vi "WinCI Run Provider.vi"(8 "error in (no error)":errorcluster) -> (0 "error out":errorcluster)   [LabVIEW 2017, in "NI_SCC_WinCI.lvlib"]
uses:
  <vilib>/SourceControl/Providers/WinCI/NI_SCC_WinCI.lvlib
  <vilib>/SourceControl/support/SCCSup Message Strings GLBL.vi
panel:
  out "result":i32
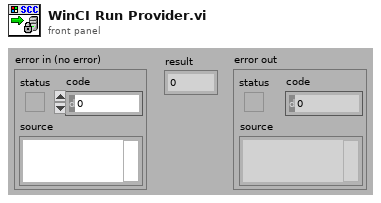
[diagram p1: front panel]
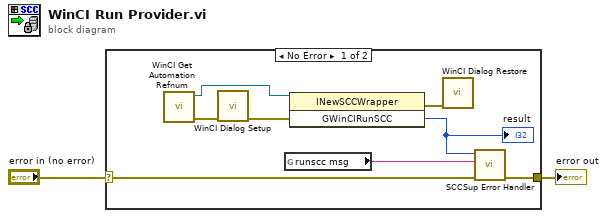
[diagram p0: block diagram]
diagram:
  n1 = case shown="No Error" "error in (no error)" {
    selector: "error in (no error)" -> [w9 w11]
    tunnel: [w10 w11] -> w1
    frame No Error {
      n2 = call <vilib>:"WinCI Get Automation Refnum.vi"() -> ("error out"=w5:errorcluster, "automation refnum"=w6:refnum<k7>)  [unwired: 10 out]
      n3 = call <vilib>:"WinCI Dialog Setup.vi"("error in"=w5) -> ("error out"=w4:errorcluster)  [unwired: 10 out]
      n4 = global read "SCCSup Message Strings GLBL.vi" "runscc msg"() -> (w8:string)
      n5 = invoke class="INewSCCWrapper" method="GWinCIRunSCC"(reference=w6, error in=w4) -> (error out=w3:errorcluster, "GWinCIRunSCC"=w7:i32)  [unwired: 1 in, 1 out]
      "result" <- w7
      n6 = call <vilib>:"WinCI Dialog Restore.vi"("error in"=w3) -> ()  [unwired: 11 out]
      n7 = call <vilib>:"SCCSup Error Handler.vi"("error in (no error)"=w9, "operation message"=w8, "scc error code"=w7) -> ("error out"=w10:errorcluster)  [unwired: 1 in, 7 out]
    }
    frame Error {
    }
  }
  "error out" <- w1
